vi "Receive Command.vi"(8 "error in (no error)":errorcluster, 9 "timeout in ms (0)":i32 format="%d ms", 11 "Plugin Thread in":refnum<class "Plugin Thread.lvclass">) -> (0 "error out":errorcluster, 1 "timed out?":bool, 2 "command":T1={"Command"=enum."Rx", "Command Parameters"={"arg1"=0, "arg2"=0}}, 3 "Plugin Thread out":refnum<class "Plugin Thread.lvclass">)   [LabVIEW 2017, in "DSF Core.lvlib" / "Plugin Thread.lvclass"]
uses:
  Plugin Thread.lvclass
  Interfaces/Transceiver Interface/Command Data.ctl
  Interfaces/Transceiver Interface/Command.ctl
  Interfaces/Transceiver Interface/Command Parameters.ctl
  Plugin Thread.lvclass/Plugin Thread.ctl
  Interfaces/Interface/Interface.lvclass/Interface.ctl
  Debug/FIFO Flags/FIFO Flags.lvclass/FIFO Flags.ctl
  Interfaces/Transceiver Interface/Read Transceiver Command.vi
  Interfaces/Interface/Read Command.vi
  Interfaces/Interface/Get Command FIFO.vi
  Interfaces/Interface/Get Debug Flags.vi
  Interfaces/Interface/Read RT FIFO(16B).vi
  Debug/FIFO Flags/Get Infinite Timeouts.vi
  Interfaces/Transceiver Interface/Plugin Interface.lvclass
  C:/Git/DSF/Data Sharing Framework/Source/Core/Engine/Classes/Interfaces/Interface/Interface.lvclass
  Interfaces/Interface/Errors.vi
  Interfaces/Interface/Command Timeout.vi
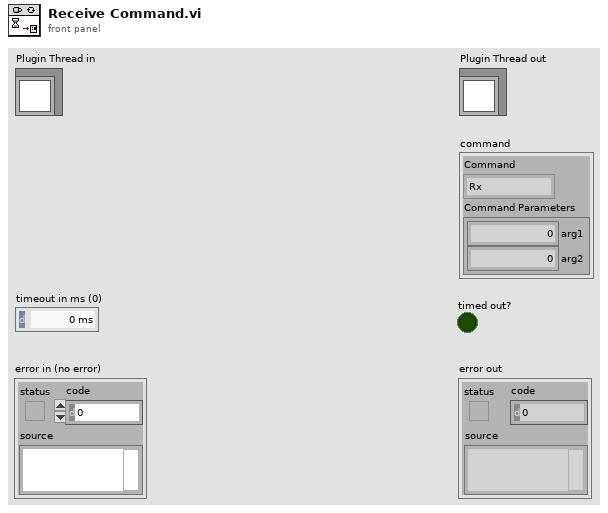
[diagram p1: front panel]
types:
  T1 = typedef "DSF Core.lvlib/Plugin Interface.lvclass/Command Data.ctl" = cluster{"Command":T2, "Command Parameters":T3}
  T2 = typedef "DSF Core.lvlib/Plugin Interface.lvclass/Command.ctl" = enum8{"Set Base Pointer", "Rx", "Tx", "Shutdown"}
  T3 = typedef "DSF Core.lvlib/Plugin Interface.lvclass/Command Parameters.ctl" = cluster{"arg1":u64, "arg2":u64}
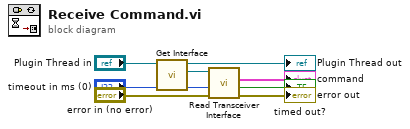
[diagram p0: block diagram]
diagram:
  n1 = call "Get Interface.vi"("Transceiver Thread in"="Plugin Thread in") -> ("Interface"=w7:refnum<class "Plugin Interface.lvclass">, "Transceiver Thread out"=→"Plugin Thread out":refnum<class "Plugin Thread.lvclass">)  [unwired: 9 in]
  n2 = call-poly "Read Transceiver Interface.vi"("error in (no error)"="error in (no error)", "timeout in ms (0)"="timeout in ms (0)", "Plugin Interface in"=w7) -> ("error out"=→"error out":errorcluster, "empty?"=→"timed out?":bool, "command"=→"command":T1)  [unwired: 4 in, 2 out]
